vi "ISMBUS_DecodeModuleCharFormat.vi"(8 "Fehler (Eingang - kein Fehler)":errorcluster, 11 "ModuleCharFormatIndex":i32) -> (0 "error (Ausgang)":errorcluster caption="Fehler  (Ausgang)", 3 "ModuleCharFormatString":string)   [LabVIEW 2016]
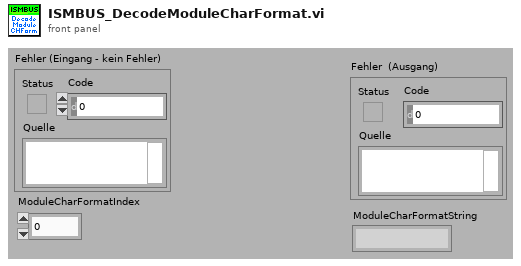
[diagram p1: front panel]
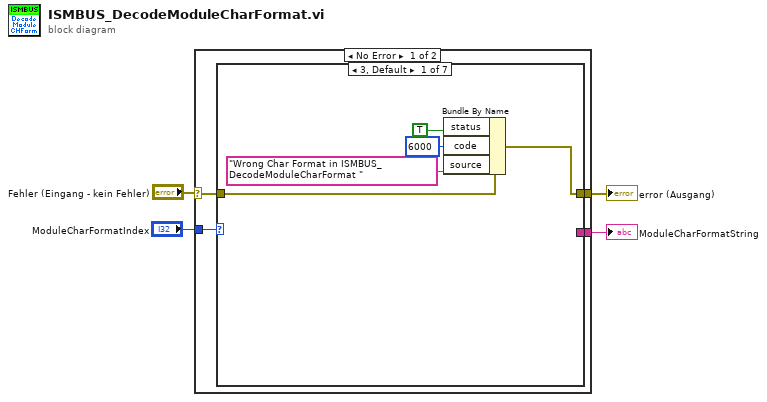
[diagram p0: block diagram]
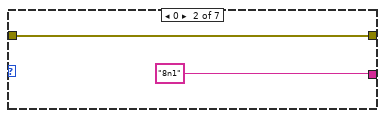
[diagram p2: hidden frame]
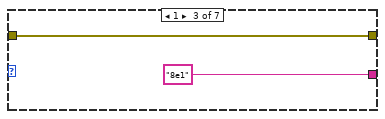
[diagram p3: hidden frame]
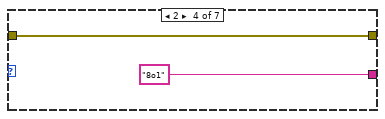
[diagram p4: hidden frame]
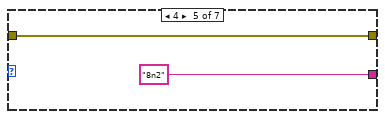
[diagram p5: hidden frame]
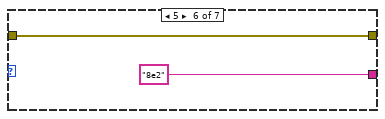
[diagram p6: hidden frame]
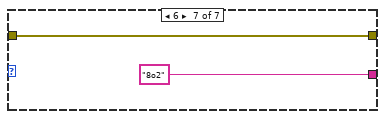
[diagram p7: hidden frame]
diagram:
  n1 = case shown="No Error" "Fehler (Eingang - kein Fehler)" {
    selector: "Fehler (Eingang - kein Fehler)" -> [w6 w26]
    tunnel: "ModuleCharFormatIndex" -> [w8 _]
    tunnel: [w7 _] -> w1
    tunnel: [w5 w26] -> w2
    frame No Error {
      n2 = case shown="3, Default" w8 {
        tunnel: [_ "8n1" "8e1" "8o1" "8n2" "8e2" "8o2"] -> w7
        tunnel: w6 -> [w12 w15 w16 w18 w20 w22 w24]
        tunnel: [w13 w15 w16 w18 w20 w22 w24] -> w5
        frame 3, Default {
          n3 = Bundle By Name(cluster=w12, "status"=TRUE, "code"=6000, "source"="Wrong Char Format in ISMBUS_DecodeModuleCharFormat ") -> (w13:errorcluster)
        }
        frame 0 {
        }
        frame 1 {
        }
        frame 2 {
        }
        frame 4 {
        }
        frame 5 {
        }
        frame 6 {
        }
      }
    }
    frame Error {
    }
  }
  "error (Ausgang)" <- w2
  "ModuleCharFormatString" <- w1
